vi "disable joystick.vi"   [LabVIEW 2014]
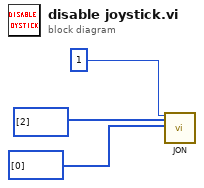
[diagram p0: block diagram]
diagram:
  n1 = call "JON.vi"("System no."=1, "JoystickID to set"=i32[] [2], "Joystick mode"=i32[] [0]) -> ()  [unwired: 15 in, 2 out]
